vi "Deadband.vi"(8 "Deadband":dbl=0.05 format="%#_13g", 11 "Input":dbl) -> (3 "f":dbl)   [LabVIEW 2018]
doc: "Implementing deadband"
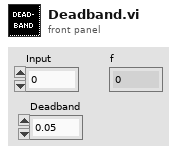
[diagram p1: front panel]
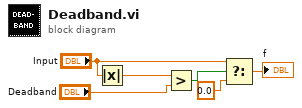
[diagram p0: block diagram]
diagram:
  n1 = Absolute Value(x="Input") -> (abs(x)=w1:dbl)
  n2 = Greater?(x=w1, y="Deadband") -> (0:w3:bool)
  n3 = Select(t="Input", s=w3, f=0.0) -> (s? t:f=→"f":dbl)
